vi "Convert Thermocouple Module to Slot Configuration.vi"(8 "error in":errorcluster, 10 "module in":refnum<class "Module.lvclass">, 11 "slot ref in":T3 format="%.0x") -> (0 "error out":errorcluster, 1 "channel measurement units":T1[](array[typedef]), 2 "channel thermocouple types":T2[](array[typedef]), 3 "slot ref out":T3 format="%.0x")   [LabVIEW 2017, in "Scan Engine Scripting.lvlib"]
doc: "Writes the channels of a thermocouple module into a system definition file’s slot configuration."
uses:
  Scan Engine Scripting.lvlib
  <vilib>/NI Veristand/Custom Device API/Custom Device Item Ref.ctl
  Modules/Module/Module.lvclass
  Modules/Channel Classes/Thermocouple Channel/Thermocouple Type.ctl
  Modules/Channel Classes/Thermocouple Channel/Measurement Units.ctl
  <vilib>/NI Veristand/Custom Device API/Custom Device API.lvlib
  Modules/Channel Classes/Thermocouple Channel/Thermocouple Channel.lvclass
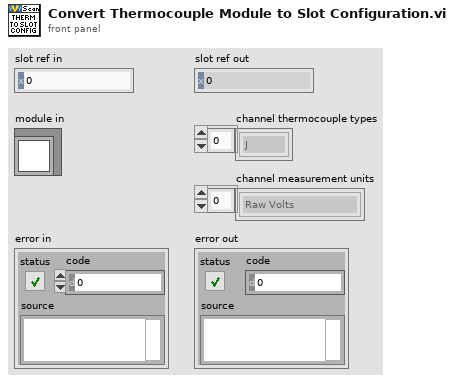
[diagram p1: front panel]
types:
  T1 = typedef "Scan Engine Scripting.lvlib/Thermocouple Channel.lvclass/Measurement Units.ctl" = enum16{"Raw Volts", "Degrees Kelvin", "Degrees Celsius", "Degrees Fahrenheit", "Degrees Rankine"}
  T2 = typedef "Scan Engine Scripting.lvlib/Thermocouple Channel.lvclass/Thermocouple Type.ctl" = enum16{"J", "K", "T", "E", "R", "S", "N", "B"}
  T3 = typedef "Custom Device API.lvlib/Custom Device Item Ref.ctl" = u64
  T4 = typedef "Scan Engine Scripting.lvlib/thermocouple channel settings.ctl" = cluster{"name":string, "default value":dbl, "thermocouple type":T2, "measurement units":T1}
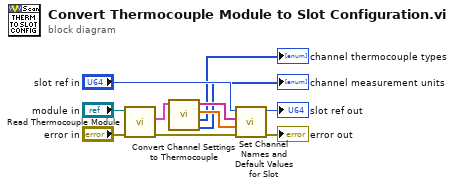
[diagram p0: block diagram]
diagram:
  n1 = call-dynamic "Read Thermocouple Module.vi"("error in"="error in", "module in"="module in") -> ("error out"=w8:errorcluster, "channel settings"=w5:T4[])  [unwired: 7 in, 1 out]
  n2 = call "Convert Channel Settings to Thermocouple.vi"("channel settings"=w5) -> ("channel measurement units"=→"channel measurement units":T1[], "channel thermocouple types"=→"channel thermocouple types":T2[], "channel default values"=w3:dbl[], "channel names"=w4:string[])  [unwired: 7 in]
  n3 = call "Set Channel Names and Default Values for Slot.vi"("error in"=w8, "default values"=w3, "channel names"=w4, "slot ref in"="slot ref in") -> ("error out"=→"error out":errorcluster, "slot ref out"=→"slot ref out":T3)  [unwired: 6 in]
